vi "Get Driver Version.vi"(8 "error in (no error)":errorcluster) -> (0 "error out":errorcluster, 3 "Instrument Driver Revision":string)   [LabVIEW 2020, in "polar_bear_plus_drivers.lvlib"]
doc: "Queries the current instrument driver version."
uses:
  <instrlib>/RxnRover/Driver Polar Bear Plus/polar_bear_plus_drivers.lvlib
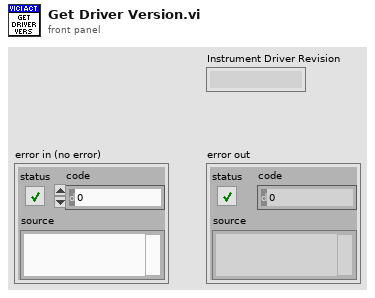
[diagram p1: front panel]
types:
  T1 = enum32{"invalid app kind", "Development System", "Run Time System", "Student Edition", "Embedded LabVIEW", "Evaluation", "Custom"}
  T2 = cluster{"Major":u16, "Minor":u16, "Fix":u16, "Build":u16}
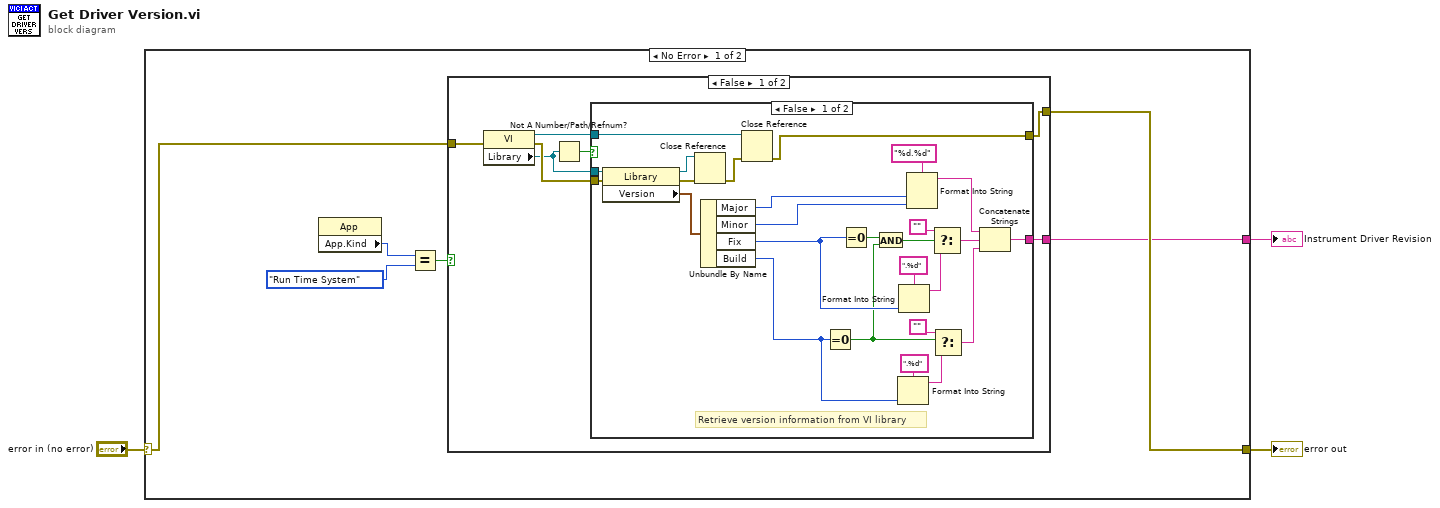
[diagram p0: block diagram]
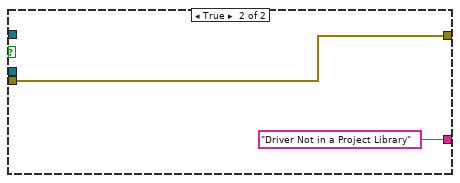
[diagram p2: hidden frame]
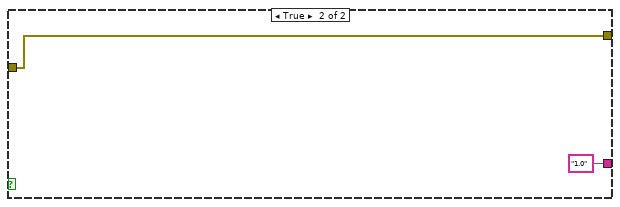
[diagram p3: hidden frame]
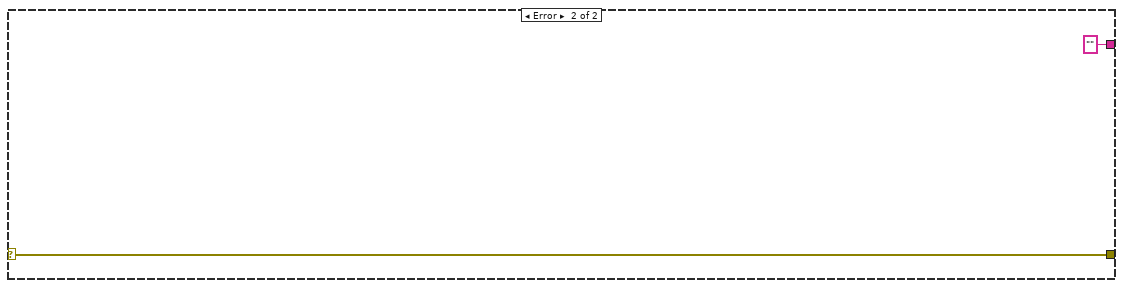
[diagram p4: hidden frame]
diagram:
  n1 = case shown="No Error" "error in (no error)" {
    selector: "error in (no error)" -> [w6 w48]
    tunnel: [w5 w48] -> w2
    tunnel: [w4 ""] -> w1
    frame No Error {
      n2 = property class="App"() -> ("App.Kind"=w8:T1)  [unwired: 2 in, 2 out]
      n3 = Equal?(x=w8, y=T1."Run Time System" ("Application:Kind")) -> (x = y?=w7:bool)
      n4 = case shown="False" w7 {
        tunnel: [w12 "1.0"] -> w4
        tunnel: w6 -> [w11 w45]
        tunnel: [w10 w45] -> w5
        frame False {
          n5 = property class="VI"(error in=w11) -> (reference out=w16:refnum<vi>, error out=w15:errorcluster, "Library"=w14:refnum<vi>)  [unwired: 1 in]
          n6 = Not A Number/Path/Refnum?(number/path/refnum=w14) -> (NaN/Path/Refnum?=w13:bool)
          n7 = case shown="False" w13 {
            tunnel: w16 -> [w39 _]
            tunnel: w15 -> [w24 w44]
            tunnel: [w19 w44] -> w10
            tunnel: [w18 "Driver Not in a Project Library"] -> w12
            tunnel: w14 -> [w17 _]
            frame False {
              # "Retrieve version information from VI library"
              n8 = property class="Library"(reference=w17, error in=w24) -> (reference out=w41:refnum<vi>, error out=w42:errorcluster, "Version"=w38:T2)
              n9 = Close Reference(reference=w41, error in (no error)=w42) -> (error out=w40:errorcluster)
              n10 = Unbundle By Name(w38) -> ("Major"=w27:u16, "Minor"=w26:u16, "Fix"=w23:u16, "Build"=w25:u16)
              n11 = Close Reference(reference=w39, error in (no error)=w40) -> (error out=w19:errorcluster)
              n12 = Equal To 0?(x=w25) -> (x = 0?=w21:bool)
              n13 = Equal To 0?(x=w23) -> (x = 0?=w22:bool)
              n14 = And(x=w22, y=w21) -> (x .and. y?=w20:bool)
              n15 = Format Into String(format string=".%d", w25) -> (resulting string=w31:string)  [unwired: 2 in, 1 out]
              n16 = Format Into String(format string=".%d", w23) -> (resulting string=w35:string)  [unwired: 2 in, 1 out]
              n17 = Format Into String(format string="%d.%d", w27, w26) -> (resulting string=w33:string)  [unwired: 2 in, 1 out]
              n18 = Select(t="", s=w20, f=w35) -> (s? t:f=w32:string)
              n19 = Select(t="", s=w21, f=w31) -> (s? t:f=w28:string)
              n20 = Concatenate Strings(w33, w32, w28) -> (w18:string)
            }
            frame True {
            }
          }
        }
        frame True {
        }
      }
    }
    frame Error {
    }
  }
  "error out" <- w2
  "Instrument Driver Revision" <- w1
